vi "VI.close_lua.vi"(5 "LuaVIEW reference":T1) -> (15 "error out":errorcluster)   [LabVIEW 2012]
doc: "Closes a VI object. This method uses the LabVIEW close reference node to release the VI reference contained in the VI object. Once closed, the VI object can no longer be used with the exception that it is allowed to call close on an already closed VI object (in which case nothing happens). This allows you to close the VI object during normal execution of the script and add a cleanup that does the same. This will cause a superfluous close attempt during normal execution without causing and error and guarantees a close when an error occurs before the in-script close is reached.\n\nWhen the VI object refers to a module, its functions are no longer callable after it is closed. When the VI is not referenced from elsewhere, it will be unloaded after being closed.\nParameters:\nobj:self, VI object to close.\nErrors:\nNot a VI object."
uses:
  typedefs/t_LuaVIEW Reference.ctl
  subvis/private/LuaVIEW Pull (object).vi
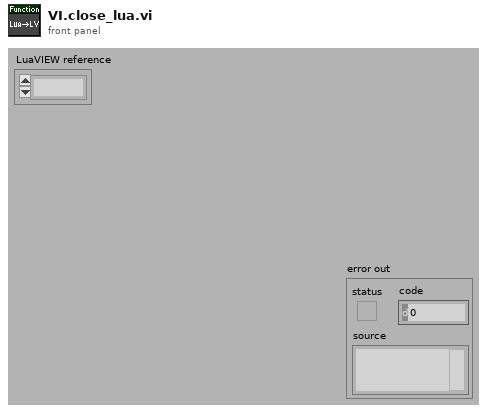
[diagram p1: front panel]
types:
  T1 = typedef "t_LuaVIEW Reference.ctl" = refnum<k1>
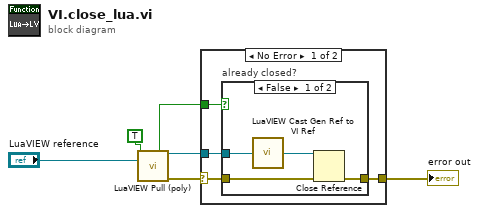
[diagram p0: block diagram]
diagram:
  n1 = call-poly "LuaVIEW Pull (poly).vi"("kill (false)"=TRUE, "LuaVIEW reference in"="LuaVIEW reference") -> ("already dead?"=w1:bool, "object refnum"=w2:refnum<vi>, "error out"=w4:errorcluster)  [unwired: 10 in, 1 out]
  n2 = case shown="No Error" w4 {
    selector: w4 -> [w9 w16]
    tunnel: [w8 w16] -> w3
    tunnel: w2 -> [w7 _]
    tunnel: w1 -> [w10 _]
    frame No Error {
      n3 = case "already closed?" shown="False" w10 {
        tunnel: w9 -> [w11 w15]
        tunnel: [w12 w15] -> w8
        tunnel: w7 -> [w14 _]
        frame False {
          n4 = call "LuaVIEW Cast Gen Ref to VI Ref.vi"("refnum in"=w14) -> ("refnum out"=w13:refnum<vi>)  [unwired: 14 in]
          n5 = Close Reference(reference=w13, error in (no error)=w11) -> (error out=w12:errorcluster)
        }
        frame True {
        }
      }
    }
    frame Error {
    }
  }
  "error out" <- w3
